vi "Forces.vi"() -> (2 "Forces":T1 {"Fz (N)" format="%.1p"; "Fy (N)" format="%.1p"; "Fx (N)" format="%.1p"})   [LabVIEW 2019]
uses:
  <userlib>/HapticSTM/HapticSTM.lvlib
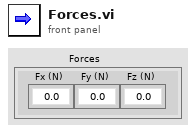
[diagram p1: front panel]
types:
  T1 = cluster{"Fx (N)":dbl, "Fy (N)":dbl, "Fz (N)":dbl}
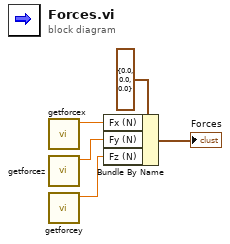
[diagram p0: block diagram]
diagram:
  n1 = call <userlib>:"getforcex.vi"() -> ("function return"=w3:dbl)  [unwired: 11 in]
  n2 = call <userlib>:"getforcez.vi"() -> ("function return"=w2:dbl)  [unwired: 11 in]
  n3 = call <userlib>:"getforcey.vi"() -> ("function return"=w1:dbl)  [unwired: 11 in]
  n4 = Bundle By Name(cluster=T1 {"Fx (N)"=0.0, "Fy (N)"=0.0, "Fz (N)"=0.0} ("Forces"), "Fx (N)"=w3, "Fy (N)"=w2, "Fz (N)"=w1) -> (→"Forces":T1)
